vi "Run Step.vi"(8 "error in (no error)":errorcluster, 10 "New Step":bool, 11 "Update Tag in":refnum<class "Update Tag Config.lvclass">) -> (0 "error out":errorcluster, 2 "Completed":bool, 3 "Update Tag out":refnum<class "Update Tag Config.lvclass">)   [LabVIEW 2015]
uses:
  Update Tag Config.lvclass
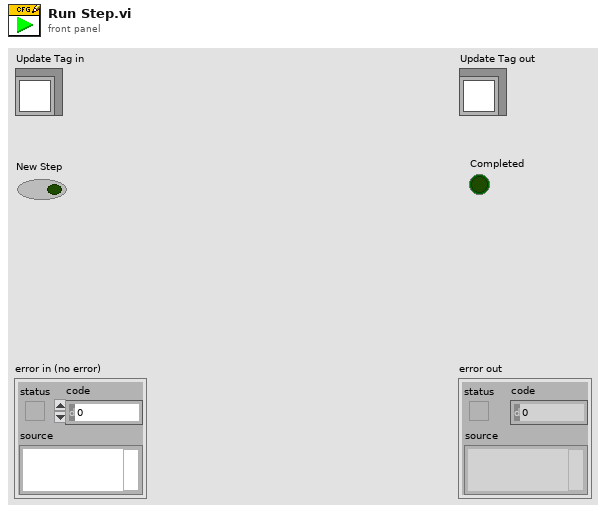
[diagram p1: front panel]
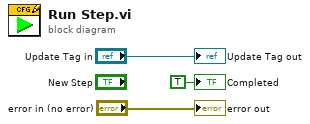
[diagram p0: block diagram]
diagram:
  "error out" <- "error in (no error)"
  "Update Tag out" <- "Update Tag in"
  "Completed" <- TRUE ("Completed")
